vi "Global 3.vi"() -> ()   [LabVIEW 2009]
panel:
  out "Shutter Status":bool caption="OK Button"
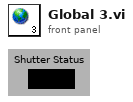
[diagram p1: front panel]
diagram:
